vi "Write RFFE_w_Repeated Waveform.vi"(5 "Num_Of_Telegrams":i32, 7 "Pins":string[](array[string])=["CLK", "SDA"], 8 "error in (no error)":errorcluster, 9 "Reg_Address_Data":T3={"Address"=81, "Data"=0} {"Address" format="%.0x"}, 10 "USID":T4 max=15, 11 "Semiconductor Module Context":T1) -> (0 "error out":errorcluster, 3 "Semiconductor Module Context Out":T1)   [LabVIEW 2013]
uses:
  <vilib>/NI_TestStand_SemiconductorModule/NI_TestStand_Semiconductor_Module.lvlibp/PinMap/General/SemiconductorModuleContext.ctl
  Controls/USID.ctl
  Controls/Reg_Address_Data.ctl
  MIPI_RFFE/Ctrls/RegReadWrite.ctl
  MIPI_RFFE/Ctrls/Configuration.ctl
  MIPI_RFFE/Ctrls/ClockDataChannels.ctl
  MIPI_RFFE/Ctrls/ExtendedRegReadWrite.ctl
  <vilib>/NI_TestStand_SemiconductorModule/NI_TestStand_Semiconductor_Module.lvlibp/PinMap/HSDIO/PinsToNIHSDIOSessions.vi
  <vilib>/Waveform/DWDTOps.llb/DWDT Append Digital Samples.vi
  <instrlib>/niHSDIO/niHSDIO.llb/niHSDIO Write Named Waveform (WDT).vi
  <vilib>/NI_TestStand_SemiconductorModule/NI_TestStand_Semiconductor_Module.lvlibp
panel:
  out "Converted Data":T2 {"Register" max=31 format="%.0x"; "Slave Address" max=15 format="%.0x"}
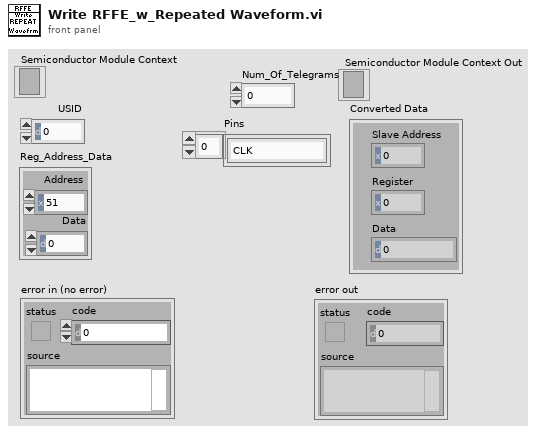
[diagram p1: front panel]
types:
  T1 = typedef "NI_TestStand_Semiconductor_Module.lvlibp/SemiconductorModuleContext.ctl" = refnum<k7>
  T2 = cluster{"Slave Address":u8, "Register":u8, "Data":u8}
  T3 = typedef "Reg_Address_Data.ctl" = cluster{"Address":u8, "Data":u8}
  T4 = typedef "USID.ctl" = u8
  T5 = typedef "Configuration.ctl" = cluster{"Samples to Allocate":i32, "Oversample Factor":u8, "Clock Channel":T6, "Data Channel":T6}
  T6 = typedef "ClockDataChannels.ctl" = enum16{"0", "1"}
  T7 = typedef "RegReadWrite.ctl" = cluster{"Slave Address":u8, "Register":u8, "Data":u8, "SetID_Pin_State":enum16{"0", "1", "Z"}}
  T8 = typedef "RFFE_Data.ctl" = cluster{"Clock Channel":T6, "Data Channel":T6, "Oversample Factor":u8, "Zero Array":u8[], "One Array":u8[], "Z Array ":u8[], "H Array":u8[], "L Array":u8[], "X Array":u8[], "Toggle (high to low)":u8[]}
  T9 = typedef "ExtendedRegReadWrite.ctl" = cluster{"Slave Address":u8, "Register":u8, "Data":u8[]}
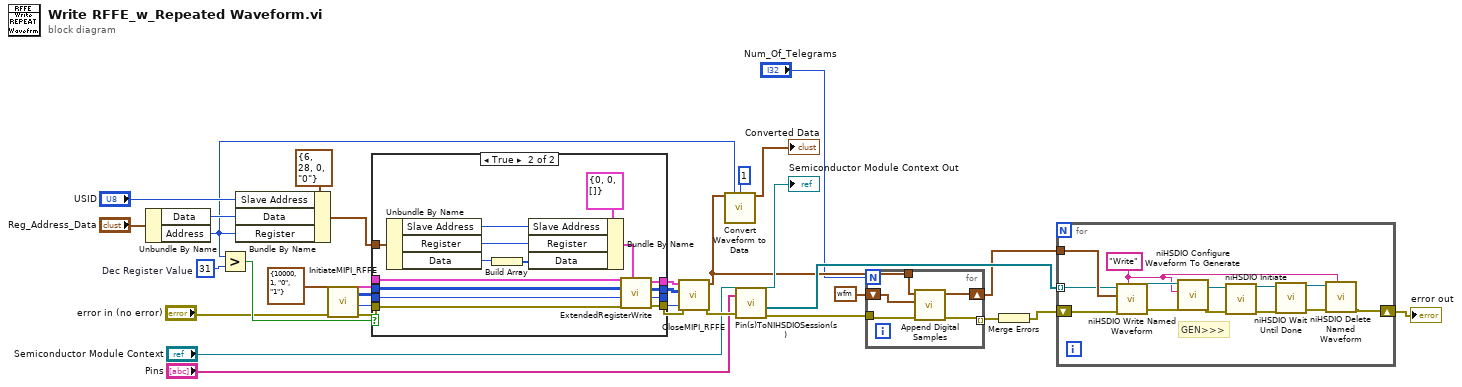
[diagram p0: block diagram]
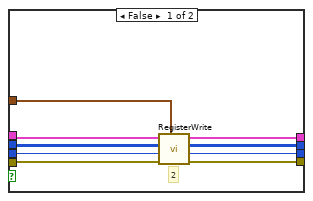
[diagram p2: hidden frame]
diagram:
  w30 = u8 31  # Dec Register Value
  n1 = Unbundle By Name("Reg_Address_Data") -> ("Data"=w12:u8, "Address"=w11:u8)
  n2 = Greater?(x=w11, y=w30) -> (0:w24:bool)
  n3 = Bundle By Name(cluster=T7 {"Slave Address"=6, "Register"=28, "Data"=0, "SetID_Pin_State"=enum."0"} ("Data"), "Slave Address"="USID", "Data"=w12, "Register"=w11) -> (w15:T7)
  n4 = call "InitiateMIPI_RFFE.vi"("error in (no error)"="error in (no error)", "Configuratation In"=T5 {"Samples to Allocate"=10000, "Oversample Factor"=1, "Clock Channel"=enum."0", "Data Channel"=enum."1"} ("Configuratation")) -> ("error out"=w23:errorcluster, "Number of Samples Out"=w22:i32, "Data Array"=w21:u8[][], "RFFE_Data"=w20:T8)  [unwired: 6 in]
  n5 = case shown="True" w24 {
    tunnel: [w37 w47] -> w29
    tunnel: [w36 w48] -> w28
    tunnel: [w35 w49] -> w27
    tunnel: [w34 w50] -> w26
    tunnel: w15 -> [w42 w56]
    tunnel: w23 -> [w38 w46]
    tunnel: w22 -> [w39 w45]
    tunnel: w21 -> [w40 w44]
    tunnel: w20 -> [w41 w43]
    frame False {
      # "2"
      n6 = call "RegisterWrite.vi"("Write Data"=w42, "error in (no error)"=w38, "Number of Samples In"=w39, "Data Array"=w40, "RFFE_Data"=w41) -> ("error out"=w34:errorcluster, "Number of Samples Out"=w35:i32, "Data Array Out"=w36:u8[][], "Configuratation Out"=w37:T8)  [unwired: 3 in]
    }
    frame True {
      n7 = Unbundle By Name(w56) -> ("Slave Address"=w55:u8, "Register"=w54:u8, "Data"=w53:u8)
      n8 = Build Array(w53) -> (w52:u8[])
      n9 = Bundle By Name(cluster=T9 {"Slave Address"=0, "Register"=0, "Data"=[]} ("Extended Read/Write"), "Slave Address"=w55, "Register"=w54, "Data"=w52) -> (w51:T9)
      n10 = call "ExtendedRegisterWrite.vi"("Extended Read/Write"=w51, "error in (no error)"=w46, "Number of Samples In"=w45, "Data Array"=w44, "RFFE_Data In"=w43) -> ("error out"=w50:errorcluster, "Number of Samples Out"=w49:i32, "Data Array Out"=w48:u8[][], "RFFE_Data Out"=w47:T8)  [unwired: 3 in]
    }
  }
  n11 = call "CloseMIPI_RFFE.vi"("error in (no error)"=w26, "Number of Samples"=w27, "Data Array"=w28, "RFFE_Data"=w29) -> ("error out"=w19:errorcluster, "Digital Waveform"=w6:digitalwaveform)  [unwired: 6 in]
  n12 = call "Convert Waveform to Data.vi"("Waveform Graph"=w6, "Register"=w11, "Ext_Read_Num_Reg"=u8 1) -> ("Converted Data"=→"Converted Data":T2)  [unwired: 10 in, 2 out]
  n13 = call-poly <vilib>:"Pin(s)ToNIHSDIOSession(s).vi"("error in (no error)"=w19, "Pins"="Pins", "Semiconductor Module Context"="Semiconductor Module Context") -> ("error out"=w3:errorcluster, "Generation Sessions"=w33:refnum<k15>[], "Semiconductor Module Context Out"=→"Semiconductor Module Context Out":T1)  [unwired: 3 in, 3 out]
  n14 = for {
    N: "Num_Of_Telegrams" -> [_]
    tunnel: w3 -> [w62]
    tunnel: [w61] -> w2 mode=indexing
    shift-right: [w60] -> w7
    shift-left: digitalwaveform {"t0"=timestamp(0 s since 1904-01-01), "dt"=0.0, "Y"={"transitions"=[], "data"=[]}} ("digital waveform out") -> [w59]
    tunnel: w6 -> [w58]
    n15 = call-poly <vilib>:"Append Digital Samples.vi"("error in (no error)"=w62, "digital waveform B"=w59, "digital waveform A"=w58) -> ("error out"=w61:errorcluster, "digital waveform out"=w60:digitalwaveform)  [unwired: 7 in]
  }
  n16 = Merge Errors(w2) -> (w1:errorcluster)
  n17 = for {
    tunnel: w33 -> [w64] mode=indexing
    shift-right: [w63] -> w31
    shift-left: w1 -> [w65]
    tunnel: w7 -> [w70]
    w66 = "Write" ("waveform name (default:\"\")")
    # "GEN>>>"
    n18 = call-poly <instrlib>:"niHSDIO Write Named Waveform.vi"("waveform name (default:\"\")"=w66, "error in (no error)"=w65, "data"=w70, "instrument handle"=w64) -> ("error out"=w73:errorcluster, "instrument handle out"=w72:refnum<k15>)  [unwired: 6 in]
    n19 = call <instrlib>:"niHSDIO Configure Waveform To Generate.vi"("error in (no error)"=w73, "waveform name"=w66, "instrument handle"=w72) -> ("error out"=w69:errorcluster, "instrument handle out"=w71:refnum<k15>)  [unwired: 7 in]
    n20 = call <instrlib>:"niHSDIO Initiate.vi"("error in (no error)"=w69, "instrument handle"=w71) -> ("error out"=w75:errorcluster, "instrument handle out"=w74:refnum<k15>)  [unwired: 8 in]
    n21 = call <instrlib>:"niHSDIO Wait Until Done.vi"("error in (no error)"=w75, "instrument handle"=w74) -> ("error out"=w68:errorcluster, "instrument handle out"=w67:refnum<k15>)  [unwired: 8 in]
    n22 = call <instrlib>:"niHSDIO Delete Named Waveform.vi"("waveform name (default:\"\")"=w66, "error in (no error)"=w68, "instrument handle"=w67) -> ("error out"=w63:errorcluster)  [unwired: 7 in, 1 out]
  }
  "error out" <- w31
